vi "16-BITSStringToBITS.vi"(11 "BITS String":string) -> (3 "BITS out":bool[](array[boolean]))   [LabVIEW 2019, in "16.lvlib"]
uses:
  16.lvlib
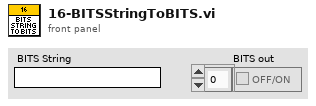
[diagram p1: front panel]
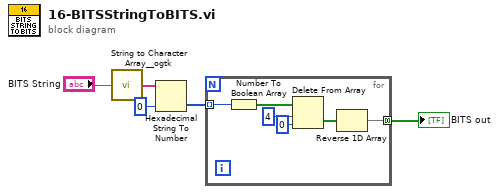
[diagram p0: block diagram]
diagram:
  n1 = call <userlib>:"String to Character Array__ogtk.vi"("Input String"="BITS String") -> ("Character Array"=w1:string[])
  n2 = Hexadecimal String To Number(string=w1, default (0uL)=u8 0 ("default (0 U32)")) -> (number=w2:u8[])  [unwired: 1 in, 1 out]
  n3 = for {
    tunnel: w2 -> [w11] mode=indexing
    tunnel: [w7] -> w4 mode=concatenating
    n4 = Number To Boolean Array(number=w11) -> (Boolean array=w10:bool[])
    n5 = Delete From Array(array=w10, length=4, index=0) -> (deleted portion=w6:bool[])  [unwired: 1 out]
    n6 = Reverse 1D Array(array=w6) -> (reversed array=w7:bool[])
  }
  "BITS out" <- w4
